vi "_AllThingsBotSpeak.vi"() -> ()   [LabVIEW 2012]
uses:
  <userlib>/BotSpeak/VIs/SubVIs/BotSpeak_Globals.vi
  <userlib>/BotSpeak/VIs/Direct/BotSpeak_Control.ctl
panel:
  out "Last Bot":T1
  out "voltage":dbl(knob) scale=-10.0..10.0
  out "State":bool
  out "value":string
  out "number":dbl
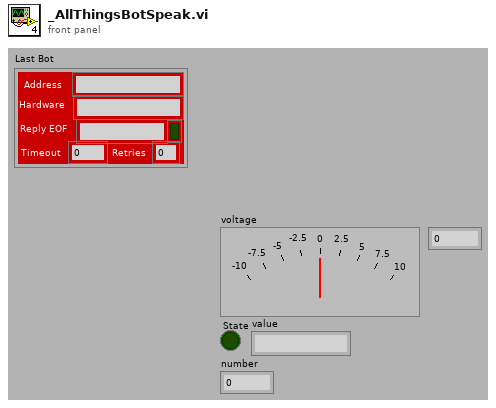
[diagram p1: front panel]
types:
  T1 = typedef "BotSpeak_Control.ctl" = cluster{"Address":string, "Reply EOF":string, "Hardware":string, "Retries":i8, "Timeout":i32, "Open?":bool}
  T2 = typedef "URAPI_Control.ctl" = cluster{"Script":string, "Whiles":u8[], "Ifs":u8[], "Supress Err":bool, "Errors":string}
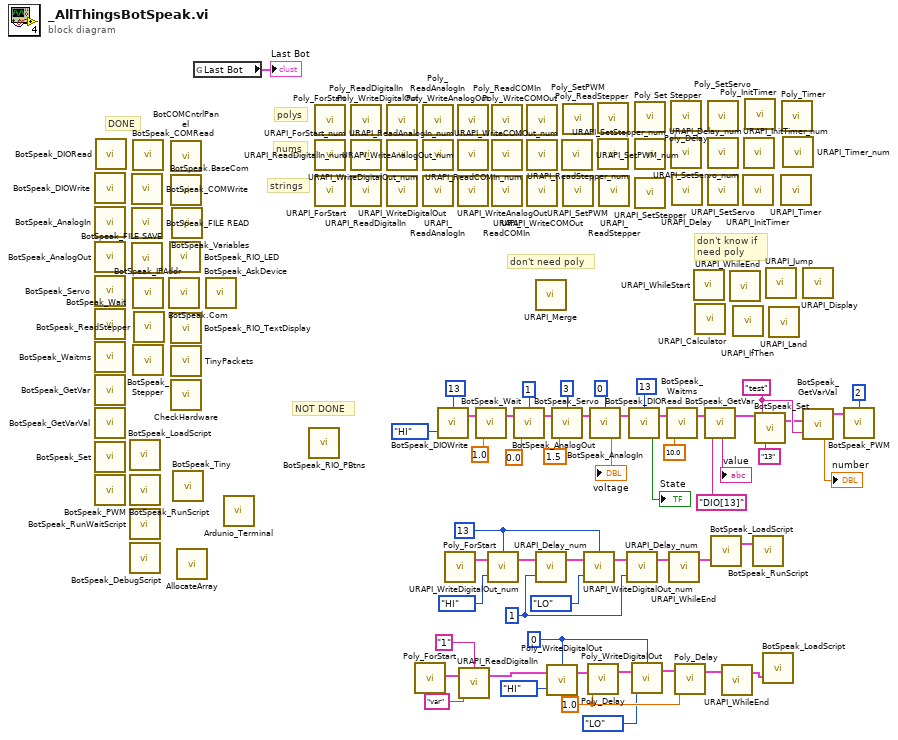
[diagram p0: block diagram]
diagram:
  w26 = "test" ("Variable In")
  w36 = sgl 1.0 ("Time In")
  w35 = u8 0 ("Channel")
  w43 = u16 1 ("Variable In")
  w48 = u8 13 ("Channel")
  # "don't know if\nneed poly"
  # "don't need poly"
  # "strings"
  # "nums"
  # "polys"
  # "NOT DONE"
  # "DONE"
  n1 = call <userlib>:"BotSpeak_DIOWrite.vi"() -> ()  [unwired: 3 in, 2 out]
  n2 = call <userlib>:"BotSpeak_AnalogIn.vi"() -> ()  [unwired: 3 in, 2 out]
  n3 = call <userlib>:"BotSpeak_AnalogOut.vi"() -> ()  [unwired: 3 in, 2 out]
  n4 = call <userlib>:"BotSpeak_Servo.vi"() -> ()  [unwired: 3 in, 2 out]
  n5 = call <userlib>:"BotSpeak_Wait.vi"() -> ()  [unwired: 3 in, 1 out]
  n6 = call <userlib>:"BotSpeak_Waitms.vi"() -> ()  [unwired: 3 in, 1 out]
  n7 = call <userlib>:"BotSpeak_GetVar.vi"() -> ()  [unwired: 2 in, 2 out]
  n8 = call <userlib>:"BotSpeak_GetVarVal.vi"() -> ()  [unwired: 3 in, 2 out]
  n9 = call <userlib>:"BotSpeak_Set.vi"() -> ()  [unwired: 3 in, 2 out]
  n10 = call <userlib>:"BotSpeak_PWM.vi"() -> ()  [unwired: 3 in, 2 out]
  n11 = call <userlib>:"BotSpeak_DIORead.vi"() -> ()  [unwired: 3 in, 2 out]
  n12 = call <userlib>:"BotSpeak_LoadScript.vi"() -> ()  [unwired: 2 in, 2 out]
  n13 = call <userlib>:"BotSpeak_RunScript.vi"() -> ()  [unwired: 2 in, 2 out]
  n14 = call <userlib>:"BotSpeak_RunWaitScript.vi"() -> ()  [unwired: 2 in, 2 out]
  n15 = call <userlib>:"BotSpeak_DebugScript.vi"() -> ()  [unwired: 2 in, 2 out]
  n16 = call <userlib>:"BotSpeak_COMWrite.vi"() -> ()  [unwired: 3 in, 2 out]
  n17 = call <userlib>:"BotSpeak_FILE READ.vi"() -> ()  [unwired: 3 in, 2 out]
  n18 = call <userlib>:"BotSpeak_FILE SAVE.vi"() -> ()  [unwired: 3 in, 2 out]
  n19 = call <userlib>:"BotSpeak_COMRead.vi"() -> ()  [unwired: 3 in, 2 out]
  n20 = call <userlib>:"BotSpeak_IPAddr.vi"() -> ()  [unwired: 3 in, 2 out]
  n21 = call <userlib>:"BotSpeak_Stepper.vi"() -> ()  [unwired: 3 in, 2 out]
  n22 = call <userlib>:"BotSpeak_ReadStepper.vi"() -> ()  [unwired: 3 in, 2 out]
  n23 = call <userlib>:"BotSpeak.Com.vi"() -> ()  [unwired: 3 in, 4 out]
  n24 = call <userlib>:"BotSpeak_RIO_LED.vi"() -> ()  [unwired: 3 in, 2 out]
  n25 = call <userlib>:"BotCOMCntrlPanel.vi"() -> ()  [unwired: 12 in]
  n26 = call <userlib>:"BotSpeak.BaseCom.vi"() -> ()  [unwired: 5 in, 2 out]
  n27 = call <userlib>:"BotSpeak_RIO_TextDisplay.vi"() -> ()  [unwired: 4 in, 1 out]
  n28 = call <userlib>:"TinyPackets.vi"() -> ()  [unwired: 4 in, 1 out]
  n29 = call <userlib>:"CheckHardware.vi"() -> ()  [unwired: 3 in, 1 out]
  n30 = call <userlib>:"BotSpeak_Variables.vi"() -> ()  [unwired: 3 in, 1 out]
  n31 = call <userlib>:"BotSpeak_Tiny.vi"() -> ()  [unwired: 2 in, 3 out]
  n32 = call <userlib>:"AllocateArray.vi"() -> ()  [unwired: 3 in, 1 out]
  n33 = global read "BotSpeak_Globals.vi" "Last Bot"() -> (→"Last Bot":T1)
  n34 = call <userlib>:"BotSpeak_AskDevice.vi"() -> ()  [unwired: 3 in, 1 out]
  n35 = call <userlib>:"Ardunio_Terminal.vi"() -> ()  [unwired: 12 in]
  n36 = call <userlib>:"BotSpeak_RIO_PBtns.vi"() -> ()  [unwired: 3 in, 2 out]
  n37 = call-poly <userlib>:"Poly_ForStart.vi"() -> ()  [unwired: 4 in, 2 out]
  n38 = call <userlib>:"URAPI_ForStart_num.vi"() -> ()  [unwired: 4 in, 2 out]
  n39 = call <userlib>:"URAPI_ForStart.vi"() -> ()  [unwired: 4 in, 2 out]
  n40 = call-poly <userlib>:"Poly_ReadDigitalIn.vi"() -> ()  [unwired: 4 in, 2 out]
  n41 = call <userlib>:"URAPI_ReadDigitalIn_num.vi"() -> ()  [unwired: 4 in, 2 out]
  n42 = call <userlib>:"URAPI_ReadDigitalIn.vi"() -> ()  [unwired: 4 in, 2 out]
  n43 = call-poly <userlib>:"Poly_WriteDigitalOut.vi"() -> ()  [unwired: 4 in, 2 out]
  n44 = call <userlib>:"URAPI_WriteDigitalOut_num.vi"() -> ()  [unwired: 4 in, 2 out]
  n45 = call <userlib>:"URAPI_WriteDigitalOut.vi"() -> ()  [unwired: 4 in, 2 out]
  n46 = call-poly <userlib>:"Poly_ForStart.vi"() -> ("URAPI Script Out"=w39:T2)  [unwired: 4 in, 1 out]
  n47 = call-poly <userlib>:"Poly_ReadAnalogIn.vi"() -> ()  [unwired: 4 in, 2 out]
  n48 = call <userlib>:"URAPI_ReadAnalogIn_num.vi"() -> ()  [unwired: 4 in, 2 out]
  n49 = call <userlib>:"URAPI_ReadAnalogIn.vi"() -> ()  [unwired: 4 in, 2 out]
  n50 = call <userlib>:"BotSpeak_DIOWrite.vi"("State"=enum32{"LO", "HI"}."HI", "DIO Line"=u32 13) -> ("Bot Settings"=w4:T1)  [unwired: 1 in, 1 out]
  n51 = call-poly <userlib>:"Poly_ForStart.vi"() -> ("URAPI Script Out"=w51:T2)  [unwired: 4 in, 1 out]
  n52 = call-poly <userlib>:"Poly_WriteAnalogOut.vi"() -> ()  [unwired: 4 in, 2 out]
  n53 = call <userlib>:"URAPI_WriteAnalogOut_num.vi"() -> ()  [unwired: 4 in, 2 out]
  n54 = call <userlib>:"URAPI_WriteAnalogOut.vi"() -> ()  [unwired: 4 in, 2 out]
  n55 = call <userlib>:"URAPI_ReadDigitalIn.vi"("Variable In"="var", "URAPI Script"=w39, "Channel"="1") -> ("URAPI Script"=w40:T2)  [unwired: 1 in, 1 out]
  n56 = call <userlib>:"BotSpeak_Wait.vi"("Wait (sec)"=1.0, "Bot Settings"=w4) -> ("Bot Settings"=w5:T1)  [unwired: 1 in]
  n57 = call <userlib>:"URAPI_WriteDigitalOut_num.vi"("Value"=enum16{"LO", "HI"}."HI" ("Variable In"), "URAPI Script"=w51, "Channel"=w48) -> ("URAPI Script"=w47:T2)  [unwired: 1 in, 1 out]
  n58 = call-poly <userlib>:"Poly_ReadCOMIn.vi"() -> ()  [unwired: 4 in, 2 out]
  n59 = call <userlib>:"URAPI_ReadCOMIn_num.vi"() -> ()  [unwired: 4 in, 2 out]
  n60 = call <userlib>:"URAPI_ReadCOMIn.vi"() -> ()  [unwired: 4 in, 2 out]
  n61 = call <userlib>:"BotSpeak_AnalogOut.vi"("voltage"=0.0, "Bot Settings"=w5, "DAC Channel"=u8 1) -> ("Bot Settings"=w6:T1)  [unwired: 1 out]
  n62 = call-poly <userlib>:"Poly_WriteCOMOut.vi"() -> ()  [unwired: 4 in, 2 out]
  n63 = call <userlib>:"URAPI_WriteCOMOut_num.vi"() -> ()  [unwired: 4 in, 2 out]
  n64 = call <userlib>:"URAPI_WriteCOMOut.vi"() -> ()  [unwired: 4 in, 2 out]
  n65 = call <userlib>:"URAPI_Merge.vi"() -> ()  [unwired: 5 in, 1 out]
  n66 = call <userlib>:"URAPI_Delay_num.vi"("Time In"=w43, "URAPI Script"=w47) -> ("URAPI Script out"=w44:T2)  [unwired: 3 in]
  n67 = call-poly <userlib>:"Poly_WriteDigitalOut.vi"("Value"=enum16{"LO", "HI"}."HI" ("Variable In"), "URAPI Script"=w40, "Channel"=w35) -> ("URAPI Script"=w30:T2)  [unwired: 1 in, 1 out]
  n68 = call <userlib>:"BotSpeak_Servo.vi"("Duty (msec)"=1.5, "Bot Settings"=w6, "DIO Line"=u8 3) -> ("Bot Settings 2"=w7:T1)  [unwired: 1 out]
  n69 = call <userlib>:"URAPI_SetPWM_num.vi"() -> ()  [unwired: 4 in, 2 out]
  n70 = call-poly <userlib>:"Poly_SetPWM.vi"() -> ()  [unwired: 4 in, 2 out]
  n71 = call <userlib>:"URAPI_SetPWM.vi"() -> ()  [unwired: 4 in, 2 out]
  n72 = call <userlib>:"URAPI_WriteDigitalOut_num.vi"("Value"=enum16{"LO", "HI"}."LO" ("Variable In"), "URAPI Script"=w44, "Channel"=w48) -> ("URAPI Script"=w45:T2)  [unwired: 1 in, 1 out]
  n73 = call-poly <userlib>:"Poly_Delay.vi"("Time In"=w36, "URAPI Script"=w30) -> ("URAPI Script out"=w31:T2)  [unwired: 3 in]
  n74 = call <userlib>:"BotSpeak_AnalogIn.vi"("Bot Settings"=w7, "A/D Channel"=u8 0) -> ("voltage"=→"voltage":dbl, "Bot Settings"=w8:T1)  [unwired: 1 in]
  n75 = call-poly <userlib>:"Poly_ReadStepper.vi"() -> ()  [unwired: 4 in, 2 out]
  n76 = call <userlib>:"URAPI_ReadStepper_num.vi"() -> ()  [unwired: 4 in, 2 out]
  n77 = call <userlib>:"URAPI_ReadStepper.vi"() -> ()  [unwired: 4 in, 2 out]
  n78 = call <userlib>:"URAPI_Delay_num.vi"("Time In"=w43, "URAPI Script"=w45) -> ("URAPI Script out"=w46:T2)  [unwired: 3 in]
  n79 = call <userlib>:"BotSpeak_DIORead.vi"("Bot Settings"=w8, "DIO Line"=u32 13) -> ("State"=→"State":bool, "Bot Settings out"=w9:T1)  [unwired: 1 in]
  n80 = call-poly <userlib>:"Poly_WriteDigitalOut.vi"("Value"=enum16{"LO", "HI"}."LO" ("Variable In"), "URAPI Script"=w31, "Channel"=w35) -> ("URAPI Script"=w32:T2)  [unwired: 1 in, 1 out]
  n81 = call-poly <userlib>:"Poly Set Stepper.vi"() -> ()  [unwired: 4 in, 2 out]
  n82 = call <userlib>:"URAPI_SetStepper_num.vi"() -> ()  [unwired: 4 in, 2 out]
  n83 = call <userlib>:"URAPI_SetStepper.vi"() -> ()  [unwired: 4 in, 2 out]
  n84 = call <userlib>:"BotSpeak_Waitms.vi"("Wait (ms)"=10.0, "Bot Settings"=w9) -> ("Bot Settings 2"=w10:T1)  [unwired: 1 in]
  n85 = call <userlib>:"URAPI_WhileEnd.vi"("URAPI Script"=w46) -> ("URAPI Script Out"=w52:T2)  [unwired: 4 in]
  n86 = call-poly <userlib>:"Poly_Delay.vi"() -> ()  [unwired: 5 in, 1 out]
  n87 = call <userlib>:"URAPI_Delay_num.vi"() -> ()  [unwired: 5 in, 1 out]
  n88 = call <userlib>:"URAPI_Delay.vi"() -> ()  [unwired: 5 in, 1 out]
  n89 = call-poly <userlib>:"Poly_Delay.vi"("Time In"=w36, "URAPI Script"=w32) -> ("URAPI Script out"=w37:T2)  [unwired: 3 in]
  n90 = call <userlib>:"URAPI_WhileStart.vi"() -> ()  [unwired: 4 in, 2 out]
  n91 = call <userlib>:"URAPI_Calculator.vi"() -> ()  [unwired: 4 in, 2 out]
  n92 = call <userlib>:"BotSpeak_GetVar.vi"("Variable In"="DIO[13]", "Bot Settings"=w10) -> ("value"=→"value":string, "Bot Settings out"=w23:T1)
  n93 = call-poly <userlib>:"Poly_SetServo.vi"() -> ()  [unwired: 4 in, 2 out]
  n94 = call <userlib>:"URAPI_SetServo_num.vi"() -> ()  [unwired: 4 in, 2 out]
  n95 = call <userlib>:"URAPI_SetServo.vi"() -> ()  [unwired: 4 in, 2 out]
  n96 = call <userlib>:"BotSpeak_LoadScript.vi"("URAPI Script"=w52) -> ("Bot Settings"=w53:T1)  [unwired: 1 in, 1 out]
  n97 = call <userlib>:"URAPI_WhileEnd.vi"("URAPI Script"=w37) -> ("URAPI Script Out"=w38:T2)  [unwired: 4 in]
  n98 = call <userlib>:"URAPI_WhileEnd.vi"() -> ()  [unwired: 5 in, 1 out]
  n99 = call <userlib>:"URAPI_IfThen.vi"() -> ()  [unwired: 4 in, 2 out]
  n100 = call <userlib>:"URAPI_InitTimer.vi"() -> ()  [unwired: 4 in, 2 out]
  n101 = call <userlib>:"URAPI_InitTimer_num.vi"() -> ()  [unwired: 4 in, 2 out]
  n102 = call-poly <userlib>:"Poly_InitTimer.vi"() -> ()  [unwired: 4 in, 2 out]
  n103 = call <userlib>:"BotSpeak_RunScript.vi"("Bot Settings"=w53) -> ()  [unwired: 1 in, 2 out]
  n104 = call <userlib>:"BotSpeak_Set.vi"("value"="13", "Variable In"=w26, "Bot Settings"=w23) -> ("Bot Settings"=w25:T1)  [unwired: 1 out]
  n105 = call <userlib>:"BotSpeak_LoadScript.vi"("URAPI Script"=w38) -> ()  [unwired: 1 in, 2 out]
  n106 = call <userlib>:"URAPI_Jump.vi"() -> ()  [unwired: 5 in, 1 out]
  n107 = call <userlib>:"URAPI_Land.vi"() -> ()  [unwired: 5 in, 1 out]
  n108 = call <userlib>:"URAPI_Timer.vi"() -> ()  [unwired: 4 in, 2 out]
  n109 = call-poly <userlib>:"Poly_Timer.vi"() -> ()  [unwired: 4 in, 2 out]
  n110 = call <userlib>:"URAPI_Timer_num.vi"() -> ()  [unwired: 4 in, 2 out]
  n111 = call <userlib>:"URAPI_Display.vi"() -> ()  [unwired: 4 in, 2 out]
  n112 = call <userlib>:"BotSpeak_GetVarVal.vi"("Variable In"=w26, "Bot Settings"=w25) -> ("number"=→"number":dbl, "Bot Settings out"=w28:T1)  [unwired: 1 in]
  n113 = call <userlib>:"BotSpeak_PWM.vi"("Bot Settings"=w28, "PWM Line"=u8 2 ("DIO Line")) -> ()  [unwired: 1 in, 2 out]
